vi "usrednianie.vi"(3 "Wartości":dbl[](array[numeric]), 4 "AkcjaUsredniania":T2=enum."DodajWartość", 5 "Wybór Komory":T1) -> (0 "Czy kolejka pełna?":bool, 1 "Przysp. uśrednione":i32)   [LabVIEW 2014]
uses:
  usrednianieVIs/AkcjaUsredniania.ctl
  parametryKomorVIs/WyborKomory.ctl
  usrednianieVIs/ParametryUsredniania.ctl
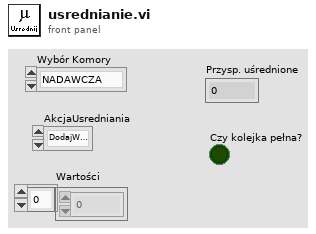
[diagram p1: front panel]
types:
  T1 = typedef "WyborKomory.ctl" = enum16{"NADAWCZA", "ODBIORCZA"}
  T2 = typedef "AkcjaUsredniania.ctl" = enum16{"Init", "DodajWartość", "OdczytajPrzyspieszenie", "WypełnijKolejkę", "Czyść"}
  T3 = typedef "ParametryUsredniania.ctl" = cluster{"Suma":dbl, "Kąty odczytane":dbl[]}
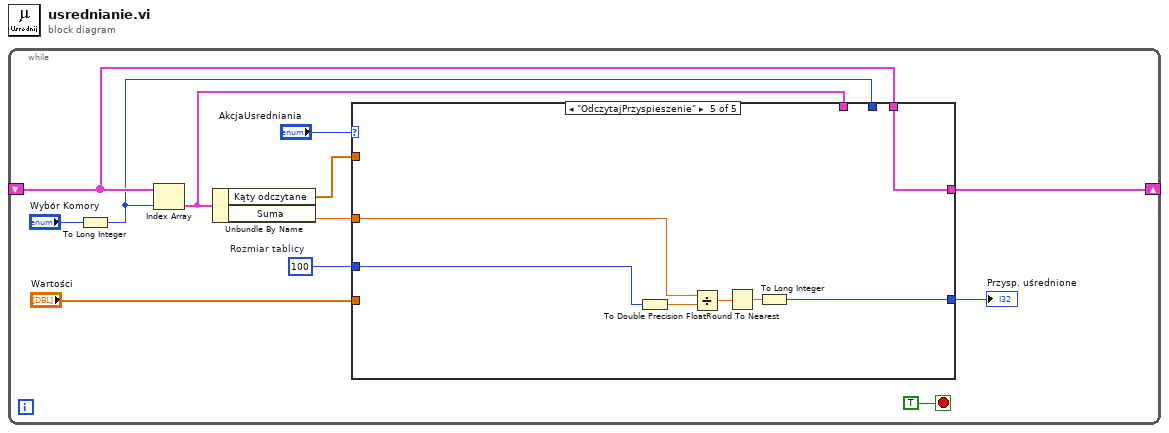
[diagram p0: block diagram]
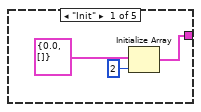
[diagram p2: hidden frame]
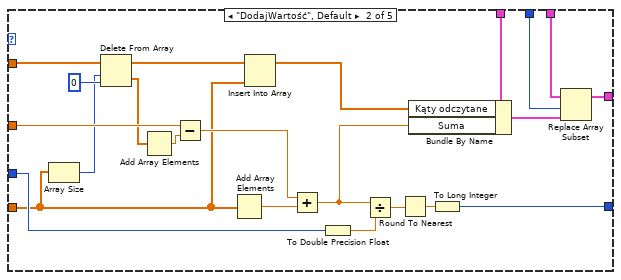
[diagram p3: hidden frame]
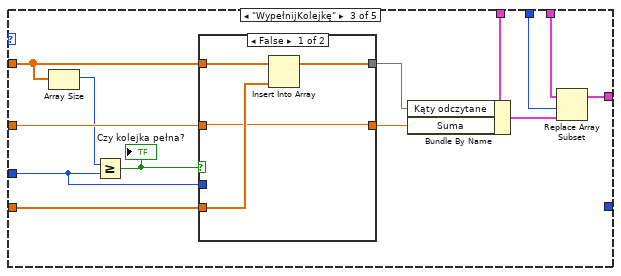
[diagram p4: hidden frame]
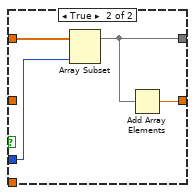
[diagram p5: hidden frame]
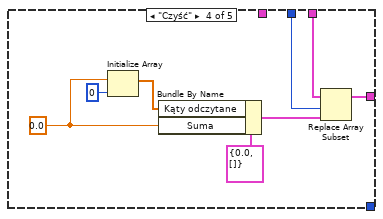
[diagram p6: hidden frame]
diagram:
  n1 = while {
    shift-right: [w11] -> _
    shift-left: _ -> [w5]
    stop <- TRUE stop-if-true
    w10 = 100  # Rozmiar tablicy
    n2 = To Long Integer(number="Wybór Komory") -> (32bit integer=w4:i32)
    n3 = Index Array(array=w5, index=w4) -> (element=w3:T3)
    n4 = Unbundle By Name(w3) -> ("Kąty odczytane"=w8:dbl[], "Suma"=w7:dbl)
    n5 = case shown="\"OdczytajPrzyspieszenie\"" "AkcjaUsredniania" {
      tunnel: w8 -> [_ w32 w47 _ _]
      tunnel: "Wartości" -> [_ w20 w48 _ _]
      tunnel: w7 -> [_ w36 w49 _ w69]
      tunnel: [w13 w25 w42 w59 w67] -> w11
      tunnel: w10 -> [_ w24 w38 _ w68]
      tunnel: w5 -> [_ w26 w41 w64 w67]
      tunnel: w4 -> [_ w27 w40 w61 _]
      tunnel: w3 -> [_ w22 w39 _ _]
      tunnel: [_ w16 _ _ w70] -> w1
      frame "Init" {
        n6 = Initialize Array(T3 {"Suma"=0.0, "Kąty odczytane"=[]} ("Parametry uśredniania"), 2 ("dimension size")) -> (w13:T3[])
      }
      frame "DodajWartość", Default {
        n7 = Array Size(array=w20) -> (size(s)=w19:i32)
        n8 = Delete From Array(array=w32, length=w19, index=0) -> (deleted portion=w18:dbl[], array with subset deleted=w31:dbl[])
        n9 = Add Array Elements(numeric array=w18) -> (sum=w17:dbl)
        n10 = Subtract(x=w36, y=w17) -> (x-y=w35:dbl)
        n11 = Add Array Elements(numeric array=w20) -> (sum=w21:dbl)
        n12 = Insert Into Array(array=w31, new element=w20) -> (w29:dbl[])  [unwired: 1 in]
        n13 = Add(x=w35, y=w21) -> (x+y=w28:dbl)
        n14 = To Double Precision Float(number=w24) -> (double precision float=w37:dbl)
        n15 = Divide(x=w28, y=w37) -> (x/y=w34:dbl)
        n16 = Round To Nearest(number=w34) -> (nearest integer value=w33:dbl)
        n17 = Bundle By Name(cluster=w22, "Kąty odczytane"=w29, "Suma"=w28) -> (w30:T3)
        n18 = To Long Integer(number=w33) -> (32bit integer=w16:i32)
        n19 = Replace Array Subset(array=w26, new element=w30, index=w27) -> (w25:T3[])
      }
      frame "WypełnijKolejkę" {
        n20 = Array Size(array=w47) -> (size(s)=w46:i32)
        n21 = Greater Or Equal?(x=w46, y=w38) -> (x >= y?=w50:bool)
        "Czy kolejka pełna?" <- w50
        n22 = case shown="False" w50 {
          tunnel: w49 -> [w51 _]
          tunnel: w48 -> [w52 _]
          tunnel: [w51 w56] -> w44
          tunnel: w47 -> [w54 w58]
          tunnel: [w53 w55] -> w45
          tunnel: w38 -> [_ w57]
          frame False {
            n23 = Insert Into Array(array=w54, new element=w52) -> (w53:dbl[])  [unwired: 1 in]
          }
          frame True {
            n24 = Array Subset(array=w58, length=w57) -> (w55:dbl[])  [unwired: 1 in]
            n25 = Add Array Elements(numeric array=w55) -> (sum=w56:dbl)
          }
        }
        n26 = Bundle By Name(cluster=w39, "Kąty odczytane"=w45, "Suma"=w44) -> (w43:T3)
        n27 = Replace Array Subset(array=w41, new element=w43, index=w40) -> (w42:T3[])
      }
      frame "Czyść" {
        w62 = 0.0 ("Wartość")
        n28 = Initialize Array(w62, 0 ("dimension size")) -> (w63:dbl[])
        n29 = Bundle By Name(cluster=T3 {"Suma"=0.0, "Kąty odczytane"=[]} ("Parametry uśredniania"), "Kąty odczytane"=w63, "Suma"=w62) -> (w65:T3)
        n30 = Replace Array Subset(array=w64, new element=w65, index=w61) -> (w59:T3[])
      }
      frame "OdczytajPrzyspieszenie" {
        n31 = To Double Precision Float(number=w68) -> (double precision float=w73:dbl)
        n32 = Divide(x=w69, y=w73) -> (x/y=w72:dbl)
        n33 = Round To Nearest(number=w72) -> (nearest integer value=w71:dbl)
        n34 = To Long Integer(number=w71) -> (32bit integer=w70:i32)
      }
    }
    "Przysp. uśrednione" <- w1
  }
